vi "Channel Data.vi"   [LabVIEW 2012]
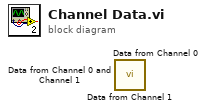
[diagram p0: block diagram]
diagram:
  n1 = call <userlib>:"Data from Channel 1.vi"() -> ()  [unwired: 11 in, 1 out]
  n2 = call <userlib>:"Data from Channel 0.vi"() -> ()  [unwired: 11 in, 1 out]
  n3 = call <userlib>:"Data from Channel 0 and Channel 1.vi"() -> ()  [unwired: 11 in, 1 out]
